vi "CANFD_Simple_Demo.vi"() -> ()   [LabVIEW 2014]
uses:
  TSMaster_API/CAN_CANFD_Function/Typedef/TLibCANFD.ctl
  <vilib>/Utility/miscctls.llb/LVPointTypeDef.ctl
  Utilities/Global/DLL_Path.vi
  Utilities/Typedef/Hardware_Subtype.ctl
  TSMaster_API/CAN_CANFD_Function/Typedef/TSCAN_CANFD_Configuration.ctl
  TSMaster_API/All_Control/Typedef/Hardware Type.ctl
panel:
  in  "DLL_Path":path=path "D:/Program Files (x86)/TOSUN/TSMaster/bin/TSMaster.dll"
  in  "Enable CH4":bool
  in  "Enable CH3":bool
  in  "Enable CH2":bool
  in  "Enable CH1":bool=TRUE
  out "Connect":bool
  in  "tab control":enum32{"CANFD1", "CANFD2", "CANFD3", "CANFD4"}(tab)
  in  "CH1  FD Frame":u8(ring) items=["Ordinary CAN Data", "FD CAN Data"]
  in  "CH1 Display Message Type":u16(ring)=1 items=["Only read received messages", "Receive&Send messages"]
  in  "CH1 Terminator":u16(ring)=1 items=["Disable", "Enable"]
  in  "CH1 Physical Channel":i32(ring) items=["CHN1", "CHN2", "CHN3", "CHN4", "CHN5", "CHN6", "CHN7", "CHN8", "CHN9", "CHN10", "CHN11", "CHN12", "CHN13", "CHN14", "CHN15", "CHN16", "CHN17", "CHN18", "CHN19", "CHN20", "CHN21", "CHN22", "CHN23", "CHN24", "CHN25", "CHN26", "CHN27", "CHN28", "CHN29", "CHN30", "CHN31", "CHN32"]
  in  "CH1 Application Logic Channel":i32(ring) items=["CHN1", "CHN2", "CHN3", "CHN4", "CHN5", "CHN6", "CHN7", "CHN8", "CHN9", "CHN10", "CHN11", "CHN12", "CHN13", "CHN14", "CHN15", "CHN16", "CHN17", "CHN18", "CHN19", "CHN20", "CHN21", "CHN22", "CHN23", "CHN24", "CHN25", "CHN26", "CHN27", "CHN28", "CHN29", "CHN30", "CHN31", "CHN32"]
  in  "CH1 Arbitration Field Baud Rate":sgl=500.0 format="%#_g k"
  in  "CH1 Data Field Baud Rate":sgl=2000.0 format="%#_g k"
  in  "CH1 Controller Type":i32(ring)=1 items=["lfdtCAN", "lfdtISOFDCAN", "lfdtNonISOFDFDCAN"]
  in  "CH1 Controller Working Mode":i32(ring) items=["lfdmNormal", "lfdmACKOff", "lfdmRestricted"]
  in  "CH1 Sending":bool
  in  "CH1ID":i32 format="%x"
  in  "CH1 Frame Format":u8(ring) items=["Standard Frame", "Extended Frame"]
  in  "CH1 Frame Type":u8(ring) items=["Data Frame", "Remote Frame", ""]
  in  "CH1SendData":u8[](array[numeric])=[0, 0, 0, 0, 0, 0, 0, 0, 0, 0, 0, 0, 0, 0, 0, 0, 0, 0, 0, 0, 0, 0, 0, 0, 0, 0, 0, 0, 0, 0, 0, 0, 0, 0, 0, 0, 0, 0, 0, 0, 0, 0, 0, 0, 0, 0, 0, 0, 0, 0, 0, 0, 0, 0, 0, 0, 0, 0, 0, 0, 0, 0, 0, 0, 0, 0, 0, 0, 0, 0, 0, 0, 0, 0, 0] format="%x"
  in  "CH1Data":i32(listbox)=-1
  in  "BRS":enum16{"Close", "Open"}(ring)
  in  "CANFD DLC":i32(ring)=15 caption="Data Length" items=["0", "1", "2", "3", "4", "5", "6", "7", "8", "12", "16", "20", "24", "32", "48", "64"]
  in  "Hardware Subtype":T1=enum."TC1016"
  in  "BRS 2":enum16{"Close", "Open"}(ring)
  in  "Hardware Subtype 2":T1=enum."TC1016"
  in  "CANFD DLC 2":i32(ring)=15 caption="Data Length" items=["0", "1", "2", "3", "4", "5", "6", "7", "8", "12", "16", "20", "24", "32", "48", "64"]
  in  "CH2  FD Frame":u8(ring) items=["Ordinary CAN Data", "FD CAN Data"]
  in  "CH2 Display Message Type":u16(ring)=1 items=["Rx", "Rx&Tx"]
  in  "CH2 Terminator":u16(ring)=1 items=["Disable", "Enable"]
  in  "CH2 Physical Channel":i32(ring)=1 items=["CHN1", "CHN2", "CHN3", "CHN4", "CHN5", "CHN6", "CHN7", "CHN8", "CHN9", "CHN10", "CHN11", "CHN12", "CHN13", "CHN14", "CHN15", "CHN16", "CHN17", "CHN18", "CHN19", "CHN20", "CHN21", "CHN22", "CHN23", "CHN24", "CHN25", "CHN26", "CHN27", "CHN28", "CHN29", "CHN30", "CHN31", "CHN32"]
  in  "CH2 Application Logic Channel":i32(ring)=1 items=["CHN1", "CHN2", "CHN3", "CHN4", "CHN5", "CHN6", "CHN7", "CHN8", "CHN9", "CHN10", "CHN11", "CHN12", "CHN13", "CHN14", "CHN15", "CHN16", "CHN17", "CHN18", "CHN19", "CHN20", "CHN21", "CHN22", "CHN23", "CHN24", "CHN25", "CHN26", "CHN27", "CHN28", "CHN29", "CHN30", "CHN31", "CHN32"]
  in  "CH2 Arbitration Field Baud Rate":sgl=500.0 format="%#_g k"
  in  "CH2 Data Field Baud Rate":sgl=2000.0 format="%#_g k"
  in  "CH2 Controller Type":i32(ring) items=["lfdtCAN", "lfdtISOFDCAN", "lfdtNonISOFDFDCAN"]
  in  "CH2 Controller Working Mode":i32(ring) items=["lfdmNormal", "lfdmACKOff", "lfdmRestricted"]
  in  "CH2 Sending":bool
  in  "CH2ID":i32 format="%x"
  in  "CH2 Frame Format":u8(ring) items=["Standard Frame", "Extended Frame"]
  in  "CH2 Frame Type":u8(ring) items=["Data Frame", "Remote Frame"]
  in  "CH2SendData":u8[](array[numeric])=[0, 0, 0, 0, 0, 0, 0, 0, 0, 0, 0, 0, 0, 0, 0, 0, 0, 0, 0, 0, 0, 0, 0, 0, 0, 0, 0, 0, 0, 0, 0, 0, 0, 0, 0, 0, 0, 0, 0, 0, 0, 0, 0, 0, 0, 0, 0, 0, 0, 0, 0, 0, 0, 0, 0, 0, 0, 0, 0, 0, 0, 0, 0, 0, 0, 0, 0, 0, 0, 0, 0, 0, 0, 0, 0, 0] format="%x"
  in  "CH2Data":i32(listbox)=-1
  in  "BRS 3":enum16{"Close", "Open"}(ring)
  in  "Hardware Subtype 3":T1=enum."TC1016"
  in  "CANFD DLC 3":i32(ring)=15 caption="Data Length" items=["0", "1", "2", "3", "4", "5", "6", "7", "8", "12", "16", "20", "24", "32", "48", "64"]
  in  "CH3 FD Frame":u8(ring) items=["Ordinary CAN Data", "FD CAN Data"]
  in  "CH3 Display Message Type":u16(ring)=1 items=["Rx", "Rx&Tx"]
  in  "CH Terminator":u16(ring)=1 items=["Disable", "Enable"]
  in  "CH3 Physical Channel":i32(ring)=2 items=["CHN1", "CHN2", "CHN3", "CHN4", "CHN5", "CHN6", "CHN7", "CHN8", "CHN9", "CHN10", "CHN11", "CHN12", "CHN13", "CHN14", "CHN15", "CHN16", "CHN17", "CHN18", "CHN19", "CHN20", "CHN21", "CHN22", "CHN23", "CHN24", "CHN25", "CHN26", "CHN27", "CHN28", "CHN29", "CHN30", "CHN31", "CHN32"]
  in  "CH3 Application Logic Channel":i32(ring)=2 items=["CHN1", "CHN2", "CHN3", "CHN4", "CHN5", "CHN6", "CHN7", "CHN8", "CHN9", "CHN10", "CHN11", "CHN12", "CHN13", "CHN14", "CHN15", "CHN16", "CHN17", "CHN18", "CHN19", "CHN20", "CHN21", "CHN22", "CHN23", "CHN24", "CHN25", "CHN26", "CHN27", "CHN28", "CHN29", "CHN30", "CHN31", "CHN32"]
  in  "CH3 Arbitration Field Baud Rate":sgl=500.0 format="%#_g k"
  in  "CH3 Data Field Baud Rate":sgl=2000.0 format="%#_g k"
  in  "CH3 Controller Type":i32(ring)=1 items=["lfdtCAN", "lfdtISOFDCAN", "lfdtNonISOFDFDCAN"]
  in  "CH3 Controller Working Mode":i32(ring) items=["lfdmNormal", "lfdmACKOff", "lfdmRestricted"]
  in  "CH3 Sending":bool
  in  "CH3ID":i32 format="%x"
  in  "CH3 Frame Format":u8(ring) items=["Standard Frame", "Extended Frame"]
  in  "CH3 Frame Type":u8(ring) items=["Data Frame", "Remote Frame"]
  in  "CH3SendData":u8[](array[numeric])=[0, 0, 0, 0, 0, 0, 0, 0, 0, 0, 0, 0, 0, 0, 0, 0, 0, 0, 0, 0, 0, 0, 0, 0, 0, 0, 0, 0, 0, 0, 0, 0, 0, 0, 0, 0, 0, 0, 0, 0, 0, 0, 0, 0, 0, 0, 0, 0, 0, 0, 0, 0, 0, 0, 0, 0, 0, 0, 0, 0, 0, 0, 0, 0, 0, 0, 0, 0, 0, 0, 0, 0, 0, 0, 0, 0] format="%x"
  in  "CH3Data":i32(listbox)=-1
  in  "BRS 4":enum16{"Close", "Open"}(ring)
  in  "Hardware Subtype 4":T1=enum."TC1016"
  in  "CANFD DLC 4":i32(ring)=15 caption="Data Length" items=["0", "1", "2", "3", "4", "5", "6", "7", "8", "12", "16", "20", "24", "32", "48", "64"]
  in  "CH4  FD Frame":u8(ring) items=["Ordinary CAN Data", "FD CAN Data"]
  in  "CH4 Display Message Type":u16(ring)=1 items=["Rx", "Rx&Tx"]
  in  "CH4 Terminator":u16(ring)=1 items=["Disable", "Enable"]
  in  "CH4 Physical Channel":i32(ring)=3 items=["CHN1", "CHN2", "CHN3", "CHN4", "CHN5", "CHN6", "CHN7", "CHN8", "CHN9", "CHN10", "CHN11", "CHN12", "CHN13", "CHN14", "CHN15", "CHN16", "CHN17", "CHN18", "CHN19", "CHN20", "CHN21", "CHN22", "CHN23", "CHN24", "CHN25", "CHN26", "CHN27", "CHN28", "CHN29", "CHN30", "CHN31", "CHN32"]
  in  "CH4 Application Logic Channel":i32(ring)=3 items=["CHN1", "CHN2", "CHN3", "CHN4", "CHN5", "CHN6", "CHN7", "CHN8", "CHN9", "CHN10", "CHN11", "CHN12", "CHN13", "CHN14", "CHN15", "CHN16", "CHN17", "CHN18", "CHN19", "CHN20", "CHN21", "CHN22", "CHN23", "CHN24", "CHN25", "CHN26", "CHN27", "CHN28", "CHN29", "CHN30", "CHN31", "CHN32"]
  in  "CH4 Arbitration Field Baud Rate":sgl=500.0 format="%#_g k"
  in  "CH4 Data Field Baud Rate":sgl=2000.0 format="%#_g k"
  in  "CH4 Controller Type":i32(ring)=1 items=["lfdtCAN", "lfdtISOFDCAN", "lfdtNonISOFDFDCAN"]
  in  "CH4 Controller Working Mode":i32(ring) items=["lfdmNormal", "lfdmACKOff", "lfdmRestricted"]
  in  "CH4 Sending":bool
  in  "CH4ID":i32 format="%x"
  in  "CH4 Frame Format":u8(ring) items=["Standard Frame", "Extended Frame"]
  in  "CH4 Frame Type":u8(ring) items=["Data Frame", "Remote Frame"]
  in  "CH4SendData":u8[](array[numeric])=[0, 0, 0, 0, 0, 0, 0, 0, 0, 0, 0, 0, 0, 0, 0, 0, 0, 0, 0, 0, 0, 0, 0, 0, 0, 0, 0, 0, 0, 0, 0, 0, 0, 0, 0, 0, 0, 0, 0, 0, 0, 0, 0, 0, 0, 0, 0, 0, 0, 0, 0, 0, 0, 0, 0, 0, 0, 0, 0, 0, 0, 0, 0, 0, 0, 0, 0, 0, 0, 0, 0, 0, 0, 0, 0, 0] format="%x"
  in  "CH4Data":i32(listbox)=-1
  in  "Number of channels used":u16(ring)=1 items=["1 Channel"=1, "2 Channels"=2, "3 Channels"=3, "4 Channels"=4, "5 Channels"=5]
  in  "Hardware on/off":bool
  in  "Exit":bool
  # "Standard Frame\nExtended Frame\nData Frame\nRemote Frame\nOrdinary CAN Data\nFD CAN Data"
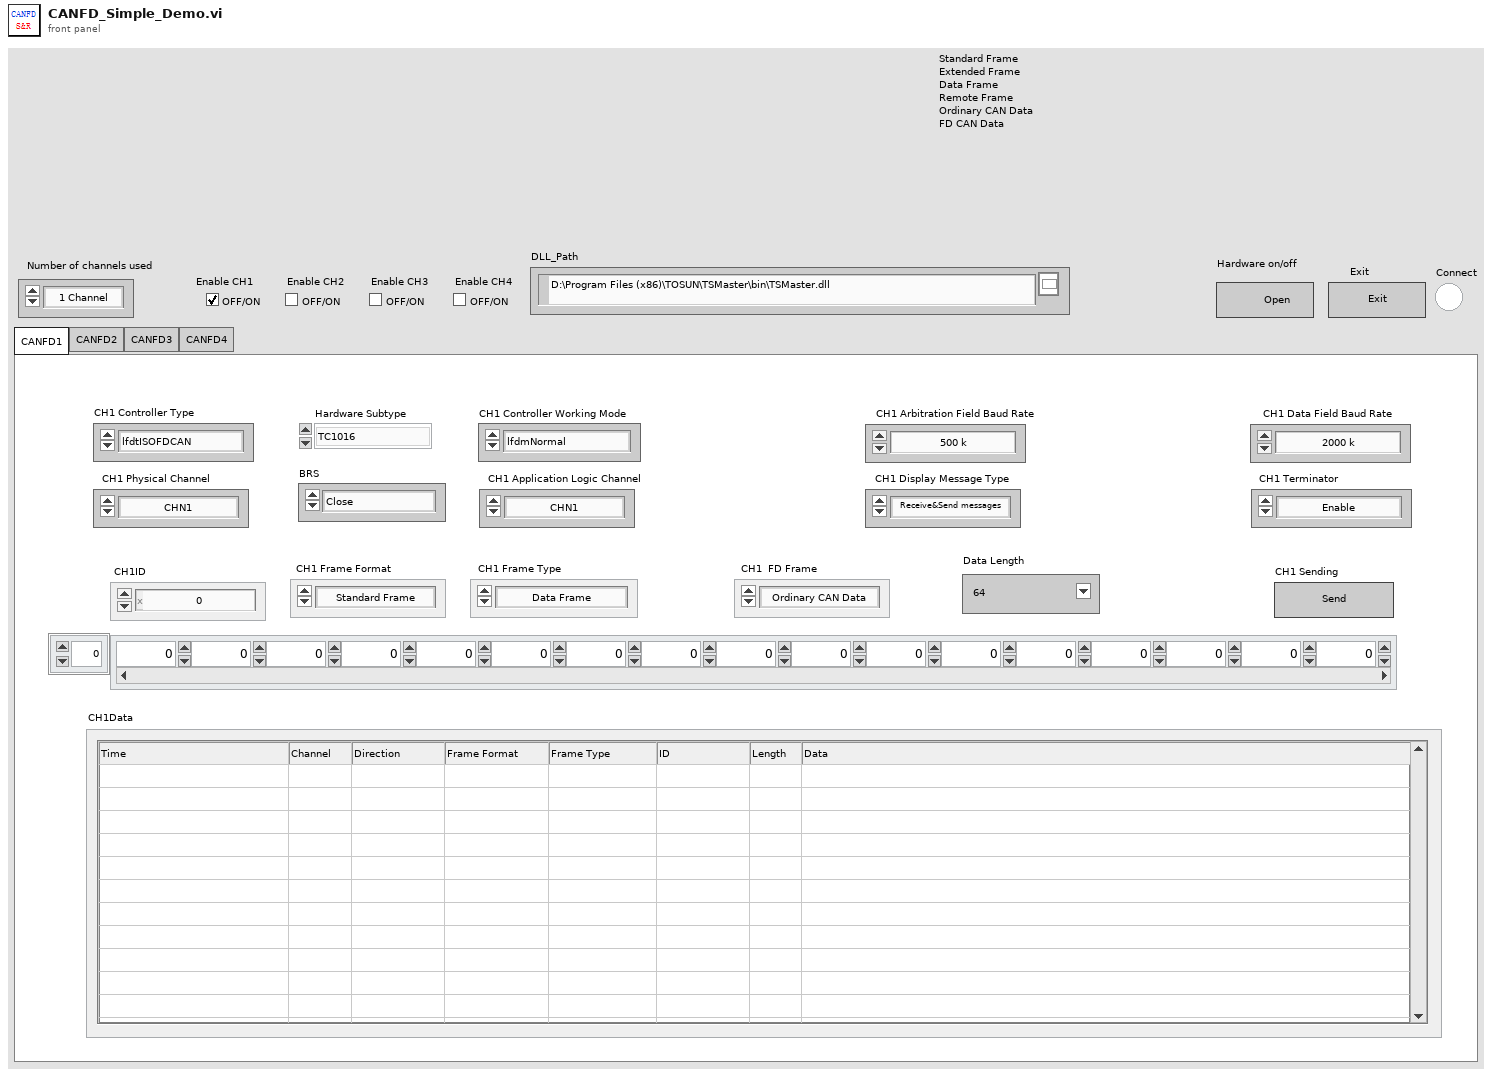
[diagram p1: front panel]
types:
  T1 = typedef "Hardware_Subtype.ctl" = enum16{"TS_UNKNOWN_DEVICE", "TSCAN_PRO", "TSCAN_Lite1", "TC1001", "TL1001", "TC1011", "TM5011", "TC1002", "TC1014", "TSCANFD2517", "TC1026", "TC1016", "TC1012", "TC1013", "TLog1002", "TC1034", "TC1018", "GW2116", "TC2115", "MP1013", "TC1113", "TC1114", "TP1013", "TC1017", "TP1018", "TF10XX", "TL1004_FD_4_LIN_2", "TE1051", "TP1051", "TP1034", "TTS9015", "TP1026", "TTS1026", "TTS1034", "TTS1018", "TL1011", "TTS1015_LiAuto", "TTS1013_LiAuto", "TTS1016Pro", "TC1054Pro", "TC1054", "TLog1038", "TO1013", "TC1034Pro", "TC1018Pro", "TC1038Pro", "TS_DEV_END"}
  T2 = typedef "LVPointTypeDef.ctl" = cluster{"Horizontal":i16, "Vertical":i16}
  T3 = cluster{"FIdxChn":u8, "FProperties":u8, "FDLC":u8, "FReserved":u8, "FIdentifier":i32, "FTimeUS":u64, "簇":cluster{"初始化的数组[0]":u8, "初始化的数组[1]":u8, "初始化的数组[2]":u8, "初始化的数组[3]":u8, "初始化的数组[4]":u8, "初始化的数组[5]":u8, "初始化的数组[6]":u8, "初始化的数组[7]":u8, "初始化的数组[8]":u8, "初始化的数组[9]":u8, "初始化的数组[10]":u8, "初始化的数组[11]":u8, "初始化的数组[12]":u8, "初始化的数组[13]":u8, "初始化的数组[14]":u8, "初始化的数组[15]":u8, "初始化的数组[16]":u8, "初始化的数组[17]":u8, "初始化的数组[18]":u8, "初始化的数组[19]":u8, "初始化的数组[20]":u8, "初始化的数组[21]":u8, "初始化的数组[22]":u8, "初始化的数组[23]":u8, "初始化的数组[24]":u8, "初始化的数组[25]":u8, "初始化的数组[26]":u8, "初始化的数组[27]":u8, "初始化的数组[28]":u8, "初始化的数组[29]":u8, "初始化的数组[30]":u8, "初始化的数组[31]":u8, "初始化的数组[32]":u8, "初始化的数组[33]":u8, "初始化的数组[34]":u8, "初始化的数组[35]":u8, "初始化的数组[36]":u8, "初始化的数组[37]":u8, "初始化的数组[38]":u8, "初始化的数组[39]":u8, "初始化的数组[40]":u8, "初始化的数组[41]":u8, "初始化的数组[42]":u8, "初始化的数组[43]":u8, "初始化的数组[44]":u8, "初始化的数组[45]":u8, "初始化的数组[46]":u8, "初始化的数组[47]":u8, "初始化的数组[48]":u8, "初始化的数组[49]":u8, "初始化的数组[50]":u8, "初始化的数组[51]":u8, "初始化的数组[52]":u8, "初始化的数组[53]":u8, "初始化的数组[54]":u8, "初始化的数组[55]":u8, "初始化的数组[56]":u8, "初始化的数组[57]":u8, "初始化的数组[58]":u8, "初始化的数组[59]":u8, "初始化的数组[60]":u8, "初始化的数组[61]":u8, "初始化的数组[62]":u8, "初始化的数组[63]":u8}}[]
  T4 = typedef "TLibCANFD.ctl" = cluster{"AIdxchn":u8, "AId":i32, "AIsStd":u8, "BRS":enum16{"Close", "Open"}, "AIsData":u8, "ADLC":i32, "AIsFD":enum16{"Classic CAN Message", "FD CAN Message"}, "FDatas":cluster{"Initialize array[0]":u8, "Initialize array[1]":u8, "Initialize array[2]":u8, "Initialize array[3]":u8, "Initialize array[4]":u8, "Initialize array[5]":u8, "Initialize array[6]":u8, "Initialize array[7]":u8, "Initialize array[8]":u8, "Initialize array[9]":u8, "Initialize array[10]":u8, "Initialize array[11]":u8, "Initialize array[12]":u8, "Initialize array[13]":u8, "Initialize array[14]":u8, "Initialize array[15]":u8, "Initialize array[16]":u8, "Initialize array[17]":u8, "Initialize array[18]":u8, "Initialize array[19]":u8, "Initialize array[20]":u8, "Initialize array[21]":u8, "Initialize array[22]":u8, "Initialize array[23]":u8, "Initialize array[24]":u8, "Initialize array[25]":u8, "Initialize array[26]":u8, "Initialize array[27]":u8, "Initialize array[28]":u8, "Initialize array[29]":u8, "Initialize array[30]":u8, "Initialize array[31]":u8, "Initialize array[32]":u8, "Initialize array[33]":u8, "Initialize array[34]":u8, "Initialize array[35]":u8, "Initialize array[36]":u8, "Initialize array[37]":u8, "Initialize array[38]":u8, "Initialize array[39]":u8, "Initialize array[40]":u8, "Initialize array[41]":u8, "Initialize array[42]":u8, "Initialize array[43]":u8, "Initialize array[44]":u8, "Initialize array[45]":u8, "Initialize array[46]":u8, "Initialize array[47]":u8, "Initialize array[48]":u8, "Initialize array[49]":u8, "Initialize array[50]":u8, "Initialize array[51]":u8, "Initialize array[52]":u8, "Initialize array[53]":u8, "Initialize array[54]":u8, "Initialize array[55]":u8, "Initialize array[56]":u8, "Initialize array[57]":u8, "Initialize array[58]":u8, "Initialize array[59]":u8, "Initialize array[60]":u8, "Initialize array[61]":u8, "Initialize array[62]":u8, "Initialize array[63]":u8}}
  T5 = cluster{"AIdxchn":u8, "AId":i32, "AIsStd":u8, "AIsData":u8, "ADLC":u8, "簇":cluster{"初始化的数组[0]":u8, "初始化的数组[1]":u8, "初始化的数组[2]":u8, "初始化的数组[3]":u8, "初始化的数组[4]":u8, "初始化的数组[5]":u8, "初始化的数组[6]":u8, "初始化的数组[7]":u8, "初始化的数组[8]":u8, "初始化的数组[9]":u8, "初始化的数组[10]":u8, "初始化的数组[11]":u8, "初始化的数组[12]":u8, "初始化的数组[13]":u8, "初始化的数组[14]":u8, "初始化的数组[15]":u8, "初始化的数组[16]":u8, "初始化的数组[17]":u8, "初始化的数组[18]":u8, "初始化的数组[19]":u8, "初始化的数组[20]":u8, "初始化的数组[21]":u8, "初始化的数组[22]":u8, "初始化的数组[23]":u8, "初始化的数组[24]":u8, "初始化的数组[25]":u8, "初始化的数组[26]":u8, "初始化的数组[27]":u8, "初始化的数组[28]":u8, "初始化的数组[29]":u8, "初始化的数组[30]":u8, "初始化的数组[31]":u8, "初始化的数组[32]":u8, "初始化的数组[33]":u8, "初始化的数组[34]":u8, "初始化的数组[35]":u8, "初始化的数组[36]":u8, "初始化的数组[37]":u8, "初始化的数组[38]":u8, "初始化的数组[39]":u8, "初始化的数组[40]":u8, "初始化的数组[41]":u8, "初始化的数组[42]":u8, "初始化的数组[43]":u8, "初始化的数组[44]":u8, "初始化的数组[45]":u8, "初始化的数组[46]":u8, "初始化的数组[47]":u8, "初始化的数组[48]":u8, "初始化的数组[49]":u8, "初始化的数组[50]":u8, "初始化的数组[51]":u8, "初始化的数组[52]":u8, "初始化的数组[53]":u8, "初始化的数组[54]":u8, "初始化的数组[55]":u8, "初始化的数组[56]":u8, "初始化的数组[57]":u8, "初始化的数组[58]":u8, "初始化的数组[59]":u8, "初始化的数组[60]":u8, "初始化的数组[61]":u8, "初始化的数组[62]":u8, "初始化的数组[63]":u8, "初始化的数组[64] ":u8}}
  T6 = cluster{"FIdxChn":u8, "FProperties":u8, "FDLC":u8, "FReserved":u8, "FIdentifier":i32, "FTimeUS":u64, "FData":cluster{"Data0":u8, "Data1":u8, "Data2":u8, "Data3":u8, "Data4":u8, "Data5":u8, "Data6":u8, "Data7":u8}}[]
  T7 = cluster{"FIdxChn":u8, "FProperties":u8, "FDLC":u8, "FReserved":u8, "FIdentifier":i32, "FTimeUS":u64, "Fdata":cluster{"初始化的数组[0]":u8, "初始化的数组[1]":u8, "初始化的数组[2]":u8, "初始化的数组[3]":u8, "初始化的数组[4]":u8, "初始化的数组[5]":u8, "初始化的数组[6]":u8, "初始化的数组[7]":u8, "初始化的数组[8]":u8, "初始化的数组[9]":u8, "初始化的数组[10]":u8, "初始化的数组[11]":u8, "初始化的数组[12]":u8, "初始化的数组[13]":u8, "初始化的数组[14]":u8, "初始化的数组[15]":u8, "初始化的数组[16]":u8, "初始化的数组[17]":u8, "初始化的数组[18]":u8, "初始化的数组[19]":u8, "初始化的数组[20]":u8, "初始化的数组[21]":u8, "初始化的数组[22]":u8, "初始化的数组[23]":u8, "初始化的数组[24]":u8, "初始化的数组[25]":u8, "初始化的数组[26]":u8, "初始化的数组[27]":u8, "初始化的数组[28]":u8, "初始化的数组[29]":u8, "初始化的数组[30]":u8, "初始化的数组[31]":u8, "初始化的数组[32]":u8, "初始化的数组[33]":u8, "初始化的数组[34]":u8, "初始化的数组[35]":u8, "初始化的数组[36]":u8, "初始化的数组[37]":u8, "初始化的数组[38]":u8, "初始化的数组[39]":u8, "初始化的数组[40]":u8, "初始化的数组[41]":u8, "初始化的数组[42]":u8, "初始化的数组[43]":u8, "初始化的数组[44]":u8, "初始化的数组[45]":u8, "初始化的数组[46]":u8, "初始化的数组[47]":u8, "初始化的数组[48]":u8, "初始化的数组[49]":u8, "初始化的数组[50]":u8, "初始化的数组[51]":u8, "初始化的数组[52]":u8, "初始化的数组[53]":u8, "初始化的数组[54]":u8, "初始化的数组[55]":u8, "初始化的数组[56]":u8, "初始化的数组[57]":u8, "初始化的数组[58]":u8, "初始化的数组[59]":u8, "初始化的数组[60]":u8, "初始化的数组[61]":u8, "初始化的数组[62]":u8, "初始化的数组[63]":u8}}[]
  T8 = typedef "TSCAN_CANFD_Configuration.ctl" = cluster{"Hardware Type":T9, "Hardware Subtype":T1, "AArbRateKbps":sgl, "AListenOnly":enum16{"Normal", "ListenOnly"}, "Int120Ohm":enum16{"Disable", "Enable"}, "EnableChannel":enum16{"Disable", "Enable"}, "AHwChannel":i32, "AAppChannel":i32, "ADataRateKbps":sgl, "AControllerType":i32, "AControllerMode":i32, "AldHW":i32}
  T9 = typedef "Hardware Type.ctl" = i32
  T10 = cluster{"CH1SendData[0]":u8, "CH1SendData[1]":u8, "CH1SendData[2]":u8, "CH1SendData[3]":u8, "CH1SendData[4]":u8, "CH1SendData[5]":u8, "CH1SendData[6]":u8, "CH1SendData[7]":u8, "CH1SendData[8]":u8, "CH1SendData[9]":u8, "CH1SendData[10]":u8, "CH1SendData[11]":u8, "CH1SendData[12]":u8, "CH1SendData[13]":u8, "CH1SendData[14]":u8, "CH1SendData[15]":u8, "CH1SendData[16]":u8, "CH1SendData[17]":u8, "CH1SendData[18]":u8, "CH1SendData[19]":u8, "CH1SendData[20]":u8, "CH1SendData[21]":u8, "CH1SendData[22]":u8, "CH1SendData[23]":u8, "CH1SendData[24]":u8, "CH1SendData[25]":u8, "CH1SendData[26]":u8, "CH1SendData[27]":u8, "CH1SendData[28]":u8, "CH1SendData[29]":u8, "CH1SendData[30]":u8, "CH1SendData[31]":u8, "CH1SendData[32]":u8, "CH1SendData[33]":u8, "CH1SendData[34]":u8, "CH1SendData[35]":u8, "CH1SendData[36]":u8, "CH1SendData[37]":u8, "CH1SendData[38]":u8, "CH1SendData[39]":u8, "CH1SendData[40]":u8, "CH1SendData[41]":u8, "CH1SendData[42]":u8, "CH1SendData[43]":u8, "CH1SendData[44]":u8, "CH1SendData[45]":u8, "CH1SendData[46]":u8, "CH1SendData[47]":u8, "CH1SendData[48]":u8, "CH1SendData[49]":u8, "CH1SendData[50]":u8, "CH1SendData[51]":u8, "CH1SendData[52]":u8, "CH1SendData[53]":u8, "CH1SendData[54]":u8, "CH1SendData[55]":u8, "CH1SendData[56]":u8, "CH1SendData[57]":u8, "CH1SendData[58]":u8, "CH1SendData[59]":u8, "CH1SendData[60]":u8, "CH1SendData[61]":u8, "CH1SendData[62]":u8, "CH1SendData[63]":u8}
  T11 = cluster{"CH2SendData[0]":u8, "CH2SendData[1]":u8, "CH2SendData[2]":u8, "CH2SendData[3]":u8, "CH2SendData[4]":u8, "CH2SendData[5]":u8, "CH2SendData[6]":u8, "CH2SendData[7]":u8, "CH2SendData[8]":u8, "CH2SendData[9]":u8, "CH2SendData[10]":u8, "CH2SendData[11]":u8, "CH2SendData[12]":u8, "CH2SendData[13]":u8, "CH2SendData[14]":u8, "CH2SendData[15]":u8, "CH2SendData[16]":u8, "CH2SendData[17]":u8, "CH2SendData[18]":u8, "CH2SendData[19]":u8, "CH2SendData[20]":u8, "CH2SendData[21]":u8, "CH2SendData[22]":u8, "CH2SendData[23]":u8, "CH2SendData[24]":u8, "CH2SendData[25]":u8, "CH2SendData[26]":u8, "CH2SendData[27]":u8, "CH2SendData[28]":u8, "CH2SendData[29]":u8, "CH2SendData[30]":u8, "CH2SendData[31]":u8, "CH2SendData[32]":u8, "CH2SendData[33]":u8, "CH2SendData[34]":u8, "CH2SendData[35]":u8, "CH2SendData[36]":u8, "CH2SendData[37]":u8, "CH2SendData[38]":u8, "CH2SendData[39]":u8, "CH2SendData[40]":u8, "CH2SendData[41]":u8, "CH2SendData[42]":u8, "CH2SendData[43]":u8, "CH2SendData[44]":u8, "CH2SendData[45]":u8, "CH2SendData[46]":u8, "CH2SendData[47]":u8, "CH2SendData[48]":u8, "CH2SendData[49]":u8, "CH2SendData[50]":u8, "CH2SendData[51]":u8, "CH2SendData[52]":u8, "CH2SendData[53]":u8, "CH2SendData[54]":u8, "CH2SendData[55]":u8, "CH2SendData[56]":u8, "CH2SendData[57]":u8, "CH2SendData[58]":u8, "CH2SendData[59]":u8, "CH2SendData[60]":u8, "CH2SendData[61]":u8, "CH2SendData[62]":u8, "CH2SendData[63]":u8}
  T12 = cluster{"CH3SendData[0]":u8, "CH3SendData[1]":u8, "CH3SendData[2]":u8, "CH3SendData[3]":u8, "CH3SendData[4]":u8, "CH3SendData[5]":u8, "CH3SendData[6]":u8, "CH3SendData[7]":u8, "CH3SendData[8]":u8, "CH3SendData[9]":u8, "CH3SendData[10]":u8, "CH3SendData[11]":u8, "CH3SendData[12]":u8, "CH3SendData[13]":u8, "CH3SendData[14]":u8, "CH3SendData[15]":u8, "CH3SendData[16]":u8, "CH3SendData[17]":u8, "CH3SendData[18]":u8, "CH3SendData[19]":u8, "CH3SendData[20]":u8, "CH3SendData[21]":u8, "CH3SendData[22]":u8, "CH3SendData[23]":u8, "CH3SendData[24]":u8, "CH3SendData[25]":u8, "CH3SendData[26]":u8, "CH3SendData[27]":u8, "CH3SendData[28]":u8, "CH3SendData[29]":u8, "CH3SendData[30]":u8, "CH3SendData[31]":u8, "CH3SendData[32]":u8, "CH3SendData[33]":u8, "CH3SendData[34]":u8, "CH3SendData[35]":u8, "CH3SendData[36]":u8, "CH3SendData[37]":u8, "CH3SendData[38]":u8, "CH3SendData[39]":u8, "CH3SendData[40]":u8, "CH3SendData[41]":u8, "CH3SendData[42]":u8, "CH3SendData[43]":u8, "CH3SendData[44]":u8, "CH3SendData[45]":u8, "CH3SendData[46]":u8, "CH3SendData[47]":u8, "CH3SendData[48]":u8, "CH3SendData[49]":u8, "CH3SendData[50]":u8, "CH3SendData[51]":u8, "CH3SendData[52]":u8, "CH3SendData[53]":u8, "CH3SendData[54]":u8, "CH3SendData[55]":u8, "CH3SendData[56]":u8, "CH3SendData[57]":u8, "CH3SendData[58]":u8, "CH3SendData[59]":u8, "CH3SendData[60]":u8, "CH3SendData[61]":u8, "CH3SendData[62]":u8, "CH3SendData[63]":u8}
  T13 = cluster{"CH4SendData[0]":u8, "CH4SendData[1]":u8, "CH4SendData[2]":u8, "CH4SendData[3]":u8, "CH4SendData[4]":u8, "CH4SendData[5]":u8, "CH4SendData[6]":u8, "CH4SendData[7]":u8, "CH4SendData[8]":u8, "CH4SendData[9]":u8, "CH4SendData[10]":u8, "CH4SendData[11]":u8, "CH4SendData[12]":u8, "CH4SendData[13]":u8, "CH4SendData[14]":u8, "CH4SendData[15]":u8, "CH4SendData[16]":u8, "CH4SendData[17]":u8, "CH4SendData[18]":u8, "CH4SendData[19]":u8, "CH4SendData[20]":u8, "CH4SendData[21]":u8, "CH4SendData[22]":u8, "CH4SendData[23]":u8, "CH4SendData[24]":u8, "CH4SendData[25]":u8, "CH4SendData[26]":u8, "CH4SendData[27]":u8, "CH4SendData[28]":u8, "CH4SendData[29]":u8, "CH4SendData[30]":u8, "CH4SendData[31]":u8, "CH4SendData[32]":u8, "CH4SendData[33]":u8, "CH4SendData[34]":u8, "CH4SendData[35]":u8, "CH4SendData[36]":u8, "CH4SendData[37]":u8, "CH4SendData[38]":u8, "CH4SendData[39]":u8, "CH4SendData[40]":u8, "CH4SendData[41]":u8, "CH4SendData[42]":u8, "CH4SendData[43]":u8, "CH4SendData[44]":u8, "CH4SendData[45]":u8, "CH4SendData[46]":u8, "CH4SendData[47]":u8, "CH4SendData[48]":u8, "CH4SendData[49]":u8, "CH4SendData[50]":u8, "CH4SendData[51]":u8, "CH4SendData[52]":u8, "CH4SendData[53]":u8, "CH4SendData[54]":u8, "CH4SendData[55]":u8, "CH4SendData[56]":u8, "CH4SendData[57]":u8, "CH4SendData[58]":u8, "CH4SendData[59]":u8, "CH4SendData[60]":u8, "CH4SendData[61]":u8, "CH4SendData[62]":u8, "CH4SendData[63]":u8}
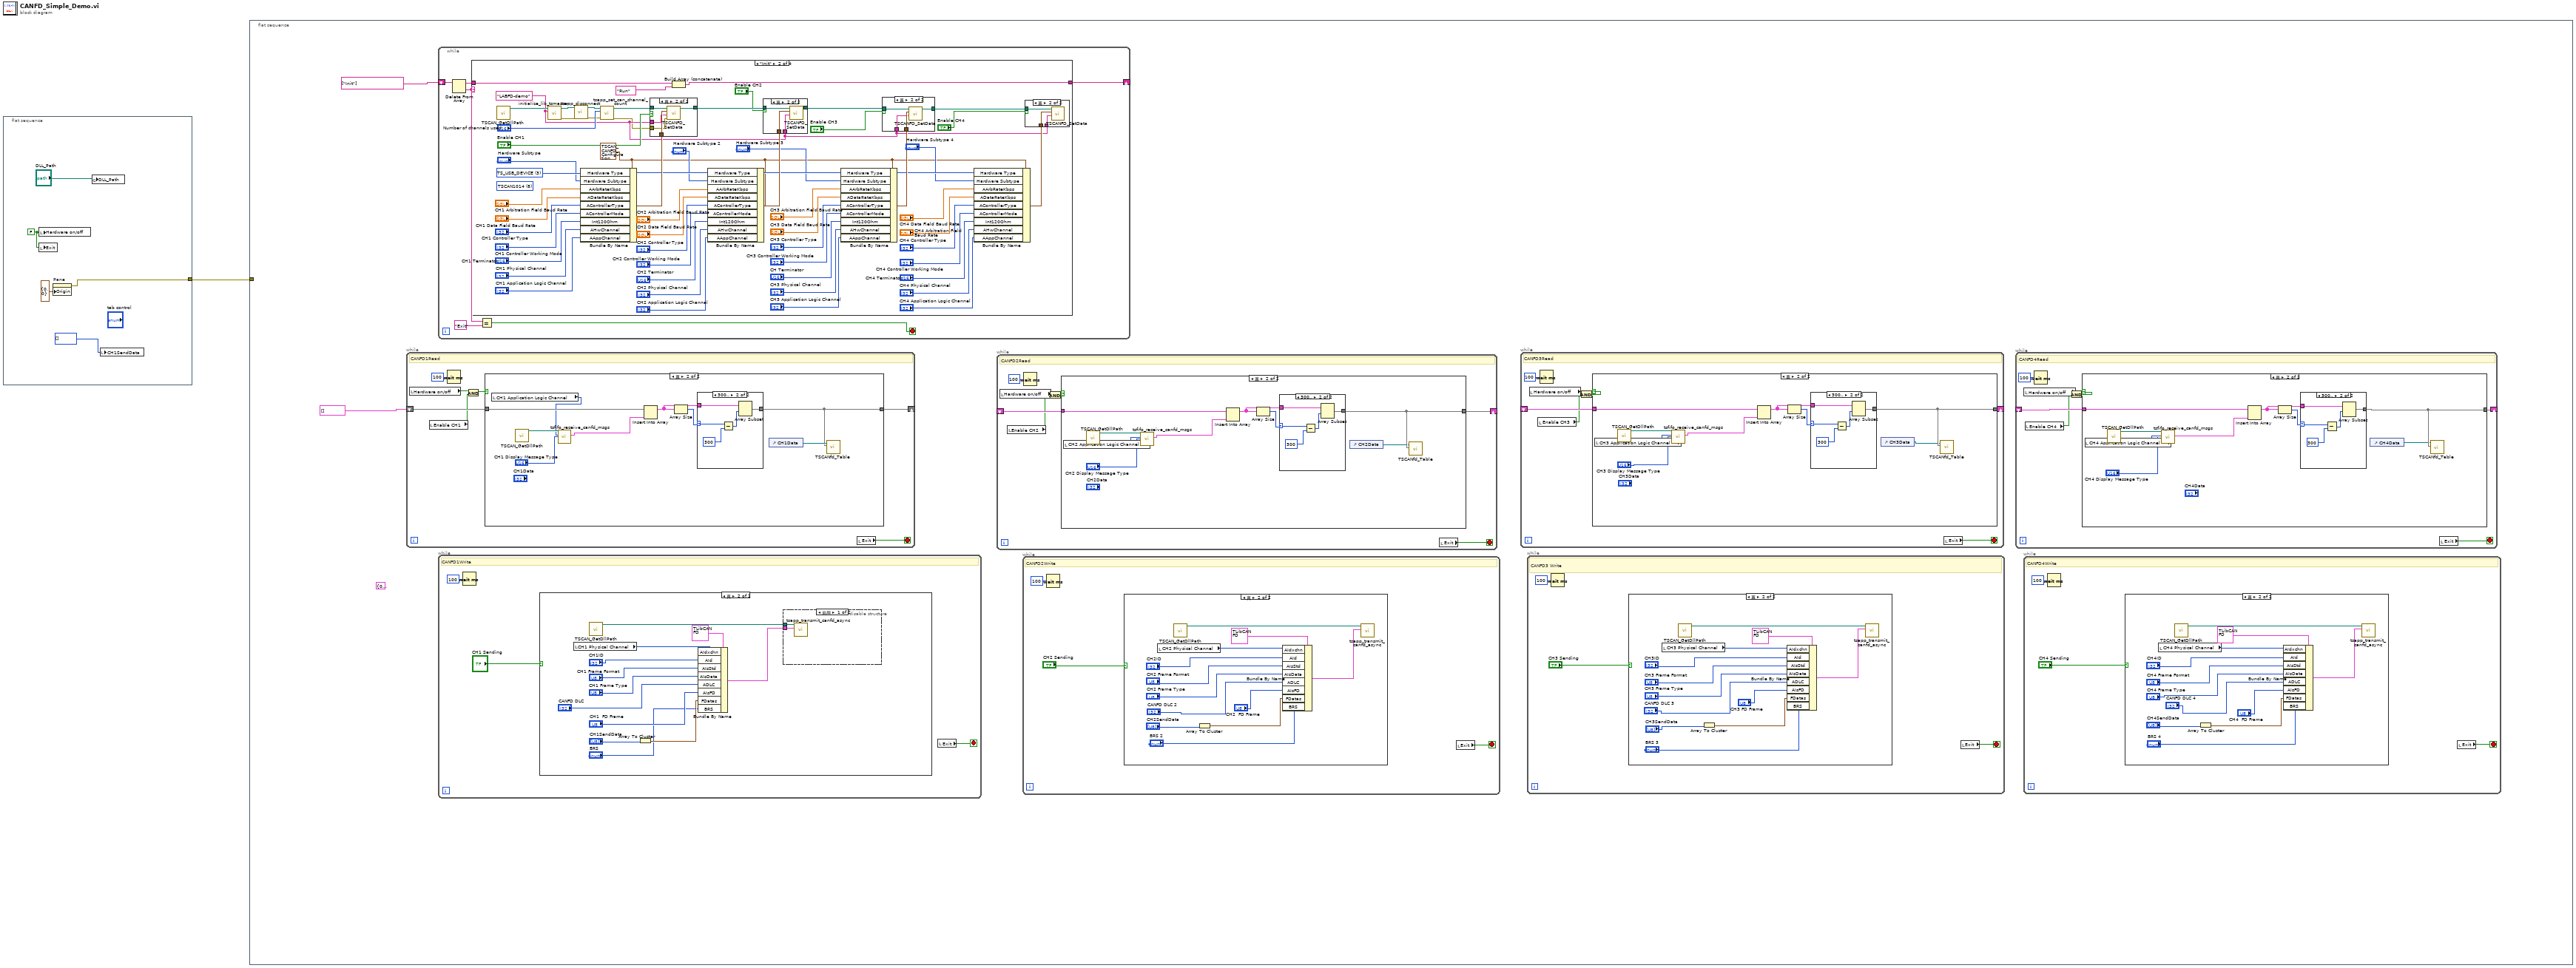
[diagram p0: block diagram]
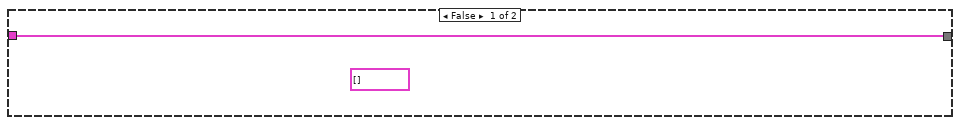
[diagram p3: hidden frame]
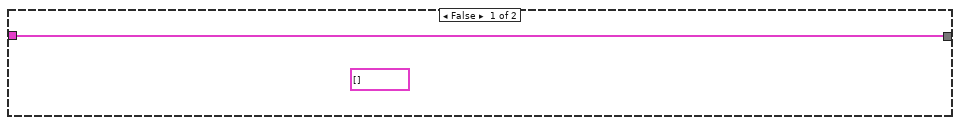
[diagram p6: hidden frame]
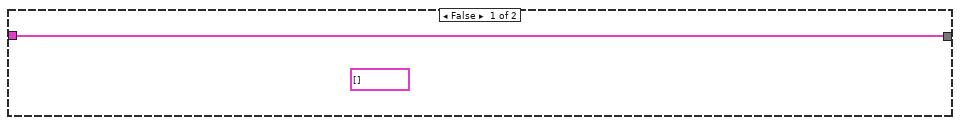
[diagram p9: hidden frame]
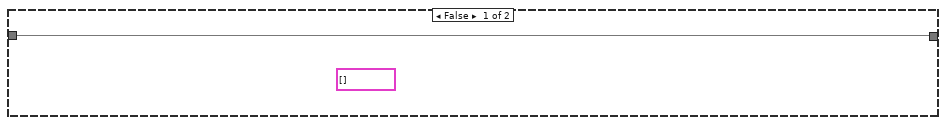
[diagram p13: hidden frame]
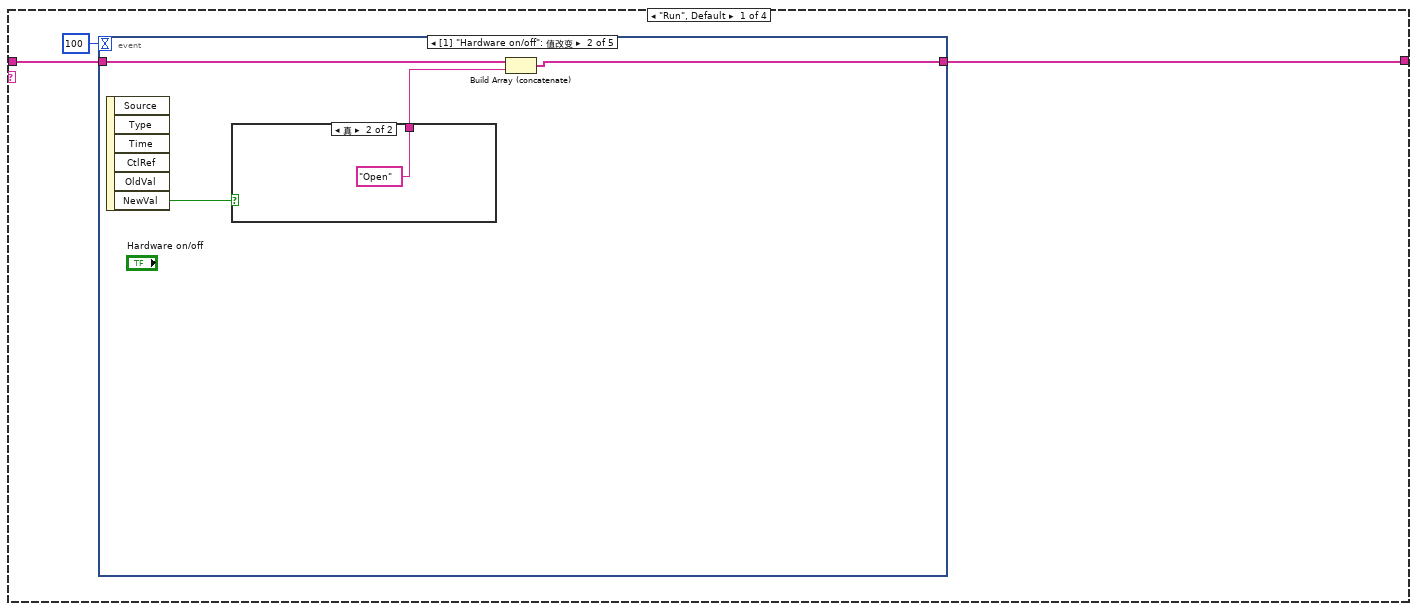
[diagram p15: hidden frame]
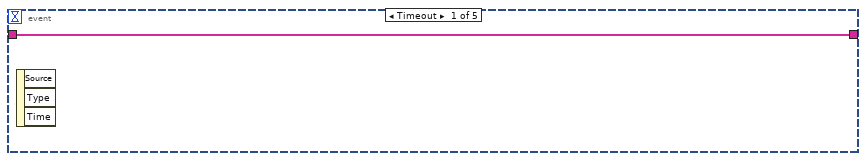
[diagram p16: hidden frame]
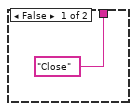
[diagram p17: hidden frame]
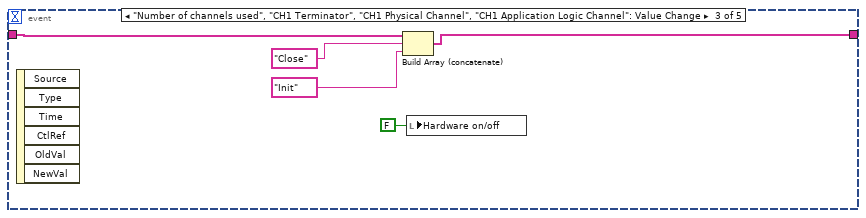
[diagram p18: hidden frame]
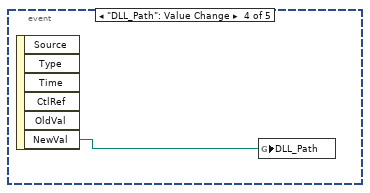
[diagram p19: hidden frame]
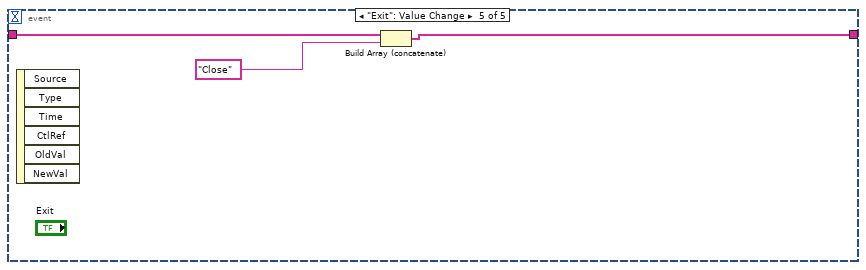
[diagram p20: hidden frame]
diagram:
  n1 = flat-sequence {
    tunnel: [w3] -> w1
    frame #0 {
      w6 = FALSE ("硬件启闭")
      n2 = local write "Hardware on/off"(w6) -> ()
      n3 = local write "Exit"(w6) -> ()
      n4 = property on="Pane" class="Pane"("Origin"=T2 {"Horizontal"=0, "Vertical"=0} ("原点")) -> (error out=w3:errorcluster)  [unwired: 2 in, 1 out]
      n5 = global write "DLL_Path.vi" "DLL_Path"("DLL_Path") -> ()
      n6 = local write "CH1SendData"(u8[] []) -> ()
    }
  }
  n7 = flat-sequence {
    tunnel: w1 -> [_]
    frame #0 {
      (unwired) T5 {"AIdxchn"=0, "AId"=0, "AIsStd"=0, "AIsData"=0, "ADLC"=0, "簇"={"初始化的数组[0]"=0, "初始化的数组[1]"=0, "初始化的数组[2]"=0, "初始化的数组[3]"=0, "初始化的数组[4]"=0, "初始化的数组[5]"=0, "初始化的数组[6]"=0, "初始化的数组[7]"=0, "初始化的数组[8]"=0, "初始化的数组[9]"=0, "初始化的数组[10]"=0, "初始化的数组[11]"=0, "初始化的数组[12]"=0, "初始化的数组[13]"=0, "初始化的数组[14]"=0, "初始化的数组[15]"=0, "初始化的数组[16]"=0, "初始化的数组[17]"=0, "初始化的数组[18]"=0, "初始化的数组[19]"=0, "初始化的数组[20]"=0, "初始化的数组[21]"=0, "初始化的数组[22]"=0, "初始化的数组[23]"=0, "初始化的数组[24]"=0, "初始化的数组[25]"=0, "初始化的数组[26]"=0, "初始化的数组[27]"=0, "初始化的数组[28]"=0, "初始化的数组[29]"=0, "初始化的数组[30]"=0, "初始化的数组[31]"=0, "初始化的数组[32]"=0, "初始化的数组[33]"=0, "初始化的数组[34]"=0, "初始化的数组[35]"=0, "初始化的数组[36]"=0, "初始化的数组[37]"=0, "初始化的数组[38]"=0, "初始化的数组[39]"=0, "初始化的数组[40]"=0, "初始化的数组[41]"=0, "初始化的数组[42]"=0, "初始化的数组[43]"=0, "初始化的数组[44]"=0, "初始化的数组[45]"=0, "初始化的数组[46]"=0, "初始化的数组[47]"=0, "初始化的数组[48]"=0, "初始化的数组[49]"=0, "初始化的数组[50]"=0, "初始化的数组[51]"=0, "初始化的数组[52]"=0, "初始化的数组[53]"=0, "初始化的数组[54]"=0, "初始化的数组[55]"=0, "初始化的数组[56]"=0, "初始化的数组[57]"=0, "初始化的数组[58]"=0, "初始化的数组[59]"=0, "初始化的数组[60]"=0, "初始化的数组[61]"=0, "初始化的数组[62]"=0, "初始化的数组[63]"=0, "初始化的数组[64] "=0}} ("TCAN 2")
      n8 = while {
        shift-right: [w143] -> _
        shift-left: T3 [] ("y") -> [w144]
        stop <- w146 stop-if-true
        # "CANFD1Read"
        n9 = local read "Hardware on/off"() -> (w142:bool)
        n10 = local read "Enable CH1"() -> (w141:bool)
        n11 = Wait (ms)(milliseconds to wait=u32 100 ("等待时间（毫秒）")) -> ()  [unwired: 1 out]
        n12 = And(x=w142, y=w141) -> (x .and. y?=w140:bool)
        n13 = case shown="真" w140 {
          tunnel: [w147 w149] -> w143
          tunnel: w144 -> [w147 w156]
          frame False {
            (unwired) T6 [] ("数组")
          }
          frame True {
            n14 = local read "CH1 Application Logic Channel"() -> (w152:i32)
            n15 = call "TSCAN_GetDllPath.vi"() -> ("DllPath"=w153:path)  [unwired: 11 in]
            n16 = call "tsfifo_receive_canfd_msgs.vi"("Display message type"="CH1 Display Message Type", "AAPPChannel"=w152, "Path"=w153) -> ("ACANMsgBuffer"=w148:T7)  [unwired: 4 in, 3 out]
            n17 = Insert Into Array(array=w156, new element=w148) -> (w154:T3)  [unwired: 1 in]
            n18 = Array Size(array=w154) -> (size(s)=w155:i32)
            n19 = case shown="300.." w155 {
              selector: w155 -> [_ w162]
              tunnel: [w157 w160] -> w149
              tunnel: w154 -> [w157 w158]
              frame 0, Default {
              }
              frame 300.. {
                n20 = Subtract(x=w162, y=300) -> (x-y=w159:i32)
                n21 = Array Subset(array=w158, index=w159) -> (w160:T3)  [unwired: 1 in]
              }
            }
            n22 = control-ref of="CH1Data"() -> (w150:refnum<vi>)
            n23 = call "TSCANfd_Table.vi"("Messages"=w149, "MCListbox reference handle"=w150) -> ()  [unwired: 10 in]
          }
        }
        n24 = local read "Exit"() -> (w146:bool)
      }
      n25 = while {
        shift-right: [w166] -> _
        shift-left: string[] ["Init"] -> [w168]
        stop <- w163 stop-if-true
        n26 = Delete From Array(array=w168) -> (deleted portion=w165:string, array with subset deleted=w167:string[])  [unwired: 2 in]
        n27 = case shown="\"Init\"" w165 {
          tunnel: w167 -> [w170 w239 w268 w274]
          tunnel: [w169 w238 w267 w275] -> w166
          frame "Run", Default {
            n28 = event shown="[1] \"Hardware on/off\": 值改变" {
              selector: _ -> [_ _ _ _ _]
              dyn-events: _ -> [_ _ _ _ _]
              timeout: 100 -> [_ _ _ _ _]
              tunnel: w170 -> [w172 w176 w183 _ w186]
              tunnel: [w172 w175 w181 _ w185] -> w169
              event Timeout {
                n29 = event-data() -> ()  [unwired: 1 in, 3 out]
              }
              event "Hardware on/off": Value Change {
                n30 = event-data() -> ("NewVal"=w174:bool)  [unwired: 1 in, 5 out]
                n31 = case shown="真" w174 {
                  tunnel: ["Close" "Open"] -> w173
                  frame False {
                  }
                  frame True {
                  }
                }
                n32 = Build Array (concatenate)(w176, w173) -> (w175:string[])
              }
              event "Number of channels used", "CH1 Terminator", "CH1 Physical Channel", "CH1 Application Logic Channel": Value Change {
                n33 = event-data() -> ()  [unwired: 1 in, 6 out]
                n34 = Build Array (concatenate)(w183, "Close", "Init") -> (w181:string[])
                n35 = local write "Hardware on/off"(FALSE ("硬件启闭")) -> ()
              }
              event "DLL_Path": Value Change {
                n36 = event-data() -> ("NewVal"=w184:path)  [unwired: 1 in, 5 out]
                n37 = global write "DLL_Path.vi" "DLL_Path"(w184) -> ()
              }
              event "Exit": Value Change {
                n38 = event-data() -> ()  [unwired: 1 in, 6 out]
                n39 = Build Array (concatenate)(w186, "Close") -> (w185:string[])
              }
            }
          }
          frame "Init" {
            w192 = T8 {"Hardware Type"=8, "Hardware Subtype"=enum."TC1016", "AArbRateKbps"=250.0, "AListenOnly"=enum."Normal", "Int120Ohm"=enum."Enable", "EnableChannel"=enum."Enable", "AHwChannel"=0, "AAppChannel"=0, "ADataRateKbps"=250.0, "AControllerType"=0, "AControllerMode"=0, "AldHW"=0} ("CANFD Configuration")
            w191 = "LABFD-demo" ("AppName")
            (unwired) 8 items=["BUS_UNKNOWN_TYPE", "TSCAN_PRO_4", "TSCAN_LITE_2", "TSCANMini", "TSLinMini", "TSCANFDmini", "TSCAN_LIN_IO_2", "TSCAN_LITE_2", "TSCAN1014", "TSCAN_FD_Mini_1"] ("硬件型号")
            w203 = 3 items=["BUS_UNKNOWN_TYPE", "TS_TCP_DEVICE", "XL_USB_DEVICE", "TS_USB_DEVICE", "PEAK_USB_DEVICE", "KVASER_USB_DEVICE", "ZLG_USB_DEVICE", "ICS_USB_DEVICE", "TS_TC1005_DEVICE"] ("硬件类型")
            n40 = call "TSCAN_GetDllPath.vi"() -> ("DllPath"=w242:path)  [unwired: 11 in]
            n41 = call "initialize_lib_tsmaster.vi"("AppName"=w191, "Path input"=w242) -> ("error output"=w190:errorcluster, "Path output"=w243:path)  [unwired: 8 in]
            n42 = call "tsapp_disconnect.vi"("error in (no error)"=w190, "Path"=w243) -> ("error output"=w189:errorcluster, "Path output"=w244:path)  [unwired: 7 in, 1 out]
            n43 = Bundle By Name(cluster=w192, "Hardware Type"=w203, "Hardware Subtype"="Hardware Subtype", "AArbRateKbps"="CH1 Arbitration Field Baud Rate", "ADataRateKbps"="CH1 Data Field Baud Rate", "AControllerType"="CH1 Controller Type", "AControllerMode"="CH1 Controller Working Mode", "Int120Ohm"="CH1 Terminator", "AHwChannel"="CH1 Physical Channel", "AAppChannel"="CH1 Application Logic Channel") -> (w229:T8)
            n44 = call "tsapp_set_can_channel_count.vi"("error in (no error)"=w189, "Aount"="Number of channels used", "Path"=w244) -> ("error out"=w188:errorcluster, "Path output"=w237:path)  [unwired: 6 in, 1 out]
            n45 = case shown="真" "Enable CH1" {
              tunnel: w237 -> [w258 w263]
              tunnel: w229 -> [_ w262]
              tunnel: [w258 w261] -> w228
              tunnel: w191 -> [_ w260]
              tunnel: w188 -> [_ w259]
              frame False {
              }
              frame True {
                n46 = call "TSCANFD_SetData.vi"("ERROR IN"=w259, "AppName"=w260, "CANFD Configuration"=w262, "PATH"=w263) -> ("PATH OUT"=w261:path)  [unwired: 4 in, 3 out]
              }
            }
            n47 = Build Array (concatenate)(w239, "Run") -> (w238:string[])
            n48 = Bundle By Name(cluster=w192, "Hardware Type"=w203, "Hardware Subtype"="Hardware Subtype 2", "AArbRateKbps"="CH2 Arbitration Field Baud Rate", "ADataRateKbps"="CH2 Data Field Baud Rate", "AControllerType"="CH2 Controller Type", "AControllerMode"="CH2 Controller Working Mode", "Int120Ohm"="CH2 Terminator", "AHwChannel"="CH2 Physical Channel", "AAppChannel"="CH2 Application Logic Channel") -> (w224:T8)
            n49 = case shown="真" "Enable CH2" {
              tunnel: w224 -> [_ w257]
              tunnel: w228 -> [w253 w256]
              tunnel: [w253 w255] -> w216
              tunnel: w191 -> [_ w254]
              frame False {
              }
              frame True {
                n50 = call "TSCANFD_SetData.vi"("AppName"=w254, "CANFD Configuration"=w257, "PATH"=w256) -> ("PATH OUT"=w255:path)  [unwired: 5 in, 3 out]
              }
            }
            n51 = Bundle By Name(cluster=w192, "Hardware Type"=w203, "Hardware Subtype"="Hardware Subtype 3", "AArbRateKbps"="CH3 Arbitration Field Baud Rate", "ADataRateKbps"="CH3 Data Field Baud Rate", "AControllerType"="CH3 Controller Type", "AControllerMode"="CH3 Controller Working Mode", "Int120Ohm"="CH Terminator", "AHwChannel"="CH3 Physical Channel", "AAppChannel"="CH3 Application Logic Channel") -> (w213:T8)
            n52 = case shown="真" "Enable CH3" {
              tunnel: w216 -> [w248 w252]
              tunnel: [w248 w251] -> w215
              tunnel: w213 -> [_ w250]
              tunnel: w191 -> [_ w249]
              frame False {
              }
              frame True {
                n53 = call "TSCANFD_SetData.vi"("AppName"=w249, "CANFD Configuration"=w250, "PATH"=w252) -> ("PATH OUT"=w251:path)  [unwired: 5 in, 3 out]
              }
            }
            n54 = Bundle By Name(cluster=w192, "Hardware Type"=w203, "Hardware Subtype"="Hardware Subtype 4", "AArbRateKbps"="CH4 Data Field Baud Rate", "ADataRateKbps"="CH4 Arbitration Field Baud Rate", "AControllerType"="CH4 Controller Type", "AControllerMode"="CH4 Controller Working Mode", "Int120Ohm"="CH4 Terminator", "AHwChannel"="CH4 Physical Channel", "AAppChannel"="CH4 Application Logic Channel") -> (w212:T8)
            n55 = case shown="真" "Enable CH4" {
              tunnel: w212 -> [_ w247]
              tunnel: w215 -> [_ w246]
              tunnel: w191 -> [_ w245]
              frame False {
              }
              frame True {
                n56 = call "TSCANFD_SetData.vi"("AppName"=w245, "CANFD Configuration"=w247, "PATH"=w246) -> ()  [unwired: 5 in, 4 out]
              }
            }
          }
          frame "Open" {
            n57 = call "TSCAN_GetDllPath.vi"() -> ("DllPath"=w264:path)  [unwired: 11 in]
            n58 = call "tsapp_connect.vi"("Path"=w264) -> ("retuen"=w266:i32, "Path output"=w270:path)  [unwired: 8 in, 1 out]
            n59 = Build Array (concatenate)(w268, "Run") -> (w267:string[])
            n60 = Equal To 0?(x=w266) -> (x = 0?=→"Connect":bool)
            n61 = call "tsfifo_enable_receive_fifo.vi"("Path"=w270) -> ()  [unwired: 9 in, 2 out]
          }
          frame "Close" {
            n62 = call "TSCAN_GetDllPath.vi"() -> ("DllPath"=w273:path)  [unwired: 11 in]
            n63 = local write "Connect"(FALSE ("通讯")) -> ()
            n64 = call "finalize_lib_tsmaster.vi"("Path"=w273) -> ("error out"=w272:errorcluster)  [unwired: 9 in, 1 out]
            n65 = local read "Exit"() -> (w276:bool)
            n66 = case shown="假" w276 {
              tunnel: [w277 w281] -> w275
              tunnel: w274 -> [w278 w280]
              tunnel: w272 -> [_ _]
              frame False {
                n67 = Build Array (concatenate)(w278, "Run") -> (w277:string[])
              }
              frame True {
                n68 = Build Array (concatenate)(w280, "Exit") -> (w281:string[])
              }
            }
          }
        }
        n69 = Equal?(x=w165, y="Exit") -> (x = y?=w163:bool)
      }
      n70 = while {
        stop <- w125 stop-if-true
        # "CANFD1Write"
        n71 = Wait (ms)(milliseconds to wait=u32 100 ("等待时间（毫秒）")) -> ()  [unwired: 1 out]
        n72 = case shown="真" "CH1 Sending" {
          frame False {
          }
          frame True {
            n73 = local read "CH1 Physical Channel"() -> (w127:i32)
            n74 = call "TSCAN_GetDllPath.vi"() -> ("DllPath"=w131:path)  [unwired: 11 in]
            n75 = Array To Cluster(array="CH1SendData") -> (cluster=w133:T10)
            n76 = Bundle By Name(cluster=T4 {"AIdxchn"=0, "AId"=0, "AIsStd"=0, "BRS"=enum."Close", "AIsData"=0, "ADLC"=0, "AIsFD"=enum."Classic CAN Message", "FDatas"={"Initialize array[0]"=0, "Initialize array[1]"=0, "Initialize array[2]"=0, "Initialize array[3]"=0, "Initialize array[4]"=0, "Initialize array[5]"=0, "Initialize array[6]"=0, "Initialize array[7]"=0, "Initialize array[8]"=0, "Initialize array[9]"=0, "Initialize array[10]"=0, "Initialize array[11]"=0, "Initialize array[12]"=0, "Initialize array[13]"=0, "Initialize array[14]"=0, "Initialize array[15]"=0, "Initialize array[16]"=0, "Initialize array[17]"=0, "Initialize array[18]"=0, "Initialize array[19]"=0, "Initialize array[20]"=0, "Initialize array[21]"=0, "Initialize array[22]"=0, "Initialize array[23]"=0, "Initialize array[24]"=0, "Initialize array[25]"=0, "Initialize array[26]"=0, "Initialize array[27]"=0, "Initialize array[28]"=0, "Initialize array[29]"=0, "Initialize array[30]"=0, "Initialize array[31]"=0, "Initialize array[32]"=0, "Initialize array[33]"=0, "Initialize array[34]"=0, "Initialize array[35]"=0, "Initialize array[36]"=0, "Initialize array[37]"=0, "Initialize array[38]"=0, "Initialize array[39]"=0, "Initialize array[40]"=0, "Initialize array[41]"=0, "Initialize array[42]"=0, "Initialize array[43]"=0, "Initialize array[44]"=0, "Initialize array[45]"=0, "Initialize array[46]"=0, "Initialize array[47]"=0, "Initialize array[48]"=0, "Initialize array[49]"=0, "Initialize array[50]"=0, "Initialize array[51]"=0, "Initialize array[52]"=0, "Initialize array[53]"=0, "Initialize array[54]"=0, "Initialize array[55]"=0, "Initialize array[56]"=0, "Initialize array[57]"=0, "Initialize array[58]"=0, "Initialize array[59]"=0, "Initialize array[60]"=0, "Initialize array[61]"=0, "Initialize array[62]"=0, "Initialize array[63]"=0}} ("TCANFD"), "AIdxchn"=w127, "AId"="CH1ID", "AIsStd"="CH1 Frame Format", "AIsData"="CH1 Frame Type", "ADLC"="CANFD DLC", "AIsFD"="CH1  FD Frame", "FDatas"=w133, "BRS"="BRS") -> (w134:T4)
            n77 = disable-structure shown="启用" {
              disable-tunnel: w134 -> [w139 _]
              disable-tunnel: w131 -> [w138 _]
              frame Enabled {
                n78 = call "tsapp_transmit_canfd_async.vi"("TCANFD"=w139, "Path"=w138) -> ()  [unwired: 7 in, 3 out]
              }
              frame Disabled {
              }
            }
          }
        }
        n79 = local read "Exit"() -> (w125:bool)
      }
      n80 = while {
        shift-right: [w103] -> _
        shift-left: _ -> [w104]
        stop <- w106 stop-if-true
        # "CANFD2Read"
        n81 = local read "Hardware on/off"() -> (w102:bool)
        n82 = local read "Enable CH2"() -> (w100:bool)
        n83 = Wait (ms)(milliseconds to wait=u32 100 ("等待时间（毫秒）")) -> ()  [unwired: 1 out]
        n84 = And(x=w102, y=w100) -> (x .and. y?=w101:bool)
        n85 = case shown="真" w101 {
          tunnel: [w107 w112] -> w103
          tunnel: w104 -> [w107 w116]
          frame False {
            (unwired) T6 [] ("数组")
          }
          frame True {
            n86 = local read "CH2 Application Logic Channel"() -> (w110:i32)
            n87 = call "TSCAN_GetDllPath.vi"() -> ("DllPath"=w113:path)  [unwired: 11 in]
            n88 = call "tsfifo_receive_canfd_msgs.vi"("Display message type"="CH2 Display Message Type", "AAPPChannel"=w110, "Path"=w113) -> ("ACANMsgBuffer"=w108:T7)  [unwired: 4 in, 3 out]
            n89 = Insert Into Array(array=w116, new element=w108) -> (w114:T7)  [unwired: 1 in]
            n90 = Array Size(array=w114) -> (size(s)=w115:i32)
            n91 = case shown="300.." w115 {
              selector: w115 -> [_ w122]
              tunnel: [w117 w120] -> w112
              tunnel: w114 -> [w117 w118]
              frame 0, Default {
              }
              frame 300.. {
                n92 = Subtract(x=w122, y=300) -> (x-y=w119:i32)
                n93 = Array Subset(array=w118, index=w119) -> (w120:T7)  [unwired: 1 in]
              }
            }
            n94 = control-ref of="CH2Data"() -> (w111:refnum<vi>)
            n95 = call "TSCANfd_Table.vi"("Messages"=w112, "MCListbox reference handle"=w111) -> ()  [unwired: 10 in]
          }
        }
        n96 = local read "Exit"() -> (w106:bool)
      }
      n97 = while {
        stop <- w87 stop-if-true
        # "CANFD2Write"
        n98 = Wait (ms)(milliseconds to wait=u32 100 ("等待时间（毫秒）")) -> ()  [unwired: 1 out]
        n99 = case shown="真" "CH2 Sending" {
          frame False {
          }
          frame True {
            n100 = local read "CH2 Physical Channel"() -> (w98:i32)
            n101 = call "TSCAN_GetDllPath.vi"() -> ("DllPath"=w99:path)  [unwired: 11 in]
            n102 = Array To Cluster(array="CH2SendData") -> (cluster=w92:T11)
            n103 = Bundle By Name(cluster=T4 {"AIdxchn"=0, "AId"=0, "AIsStd"=0, "BRS"=enum."Close", "AIsData"=0, "ADLC"=0, "AIsFD"=enum."Classic CAN Message", "FDatas"={"Initialize array[0]"=0, "Initialize array[1]"=0, "Initialize array[2]"=0, "Initialize array[3]"=0, "Initialize array[4]"=0, "Initialize array[5]"=0, "Initialize array[6]"=0, "Initialize array[7]"=0, "Initialize array[8]"=0, "Initialize array[9]"=0, "Initialize array[10]"=0, "Initialize array[11]"=0, "Initialize array[12]"=0, "Initialize array[13]"=0, "Initialize array[14]"=0, "Initialize array[15]"=0, "Initialize array[16]"=0, "Initialize array[17]"=0, "Initialize array[18]"=0, "Initialize array[19]"=0, "Initialize array[20]"=0, "Initialize array[21]"=0, "Initialize array[22]"=0, "Initialize array[23]"=0, "Initialize array[24]"=0, "Initialize array[25]"=0, "Initialize array[26]"=0, "Initialize array[27]"=0, "Initialize array[28]"=0, "Initialize array[29]"=0, "Initialize array[30]"=0, "Initialize array[31]"=0, "Initialize array[32]"=0, "Initialize array[33]"=0, "Initialize array[34]"=0, "Initialize array[35]"=0, "Initialize array[36]"=0, "Initialize array[37]"=0, "Initialize array[38]"=0, "Initialize array[39]"=0, "Initialize array[40]"=0, "Initialize array[41]"=0, "Initialize array[42]"=0, "Initialize array[43]"=0, "Initialize array[44]"=0, "Initialize array[45]"=0, "Initialize array[46]"=0, "Initialize array[47]"=0, "Initialize array[48]"=0, "Initialize array[49]"=0, "Initialize array[50]"=0, "Initialize array[51]"=0, "Initialize array[52]"=0, "Initialize array[53]"=0, "Initialize array[54]"=0, "Initialize array[55]"=0, "Initialize array[56]"=0, "Initialize array[57]"=0, "Initialize array[58]"=0, "Initialize array[59]"=0, "Initialize array[60]"=0, "Initialize array[61]"=0, "Initialize array[62]"=0, "Initialize array[63]"=0}} ("TCANFD"), "AIdxchn"=w98, "AId"="CH2ID", "AIsStd"="CH2 Frame Format", "AIsData"="CH2 Frame Type", "ADLC"="CANFD DLC 2", "AIsFD"="CH2  FD Frame", "FDatas"=w92, "BRS"="BRS 2") -> (w88:T4)
            n104 = call "tsapp_transmit_canfd_async.vi"("TCANFD"=w88, "Path"=w99) -> ()  [unwired: 7 in, 3 out]
          }
        }
        n105 = local read "Exit"() -> (w87:bool)
      }
      n106 = while {
        shift-right: [w65] -> _
        shift-left: _ -> [w66]
        stop <- w68 stop-if-true
        # "CANFD3Read"
        n107 = local read "Hardware on/off"() -> (w64:bool)
        n108 = local read "Enable CH3"() -> (w63:bool)
        n109 = Wait (ms)(milliseconds to wait=u32 100 ("等待时间（毫秒）")) -> ()  [unwired: 1 out]
        n110 = And(x=w64, y=w63) -> (x .and. y?=w62:bool)
        n111 = case shown="真" w62 {
          tunnel: [w69 w74] -> w65
          tunnel: w66 -> [w69 w78]
          frame False {
            (unwired) T6 [] ("数组")
          }
          frame True {
            n112 = local read "CH3 Application Logic Channel"() -> (w73:i32)
            n113 = call "TSCAN_GetDllPath.vi"() -> ("DllPath"=w75:path)  [unwired: 11 in]
            n114 = call "tsfifo_receive_canfd_msgs.vi"("Display message type"="CH3 Display Message Type", "AAPPChannel"=w73, "Path"=w75) -> ("ACANMsgBuffer"=w70:T7)  [unwired: 4 in, 3 out]
            n115 = Insert Into Array(array=w78, new element=w70) -> (w76:T7)  [unwired: 1 in]
            n116 = Array Size(array=w76) -> (size(s)=w77:i32)
            n117 = case shown="300.." w77 {
              selector: w77 -> [_ w84]
              tunnel: [w79 w82] -> w74
              tunnel: w76 -> [w79 w80]
              frame 0, Default {
              }
              frame 300.. {
                n118 = Subtract(x=w84, y=300) -> (x-y=w81:i32)
                n119 = Array Subset(array=w80, index=w81) -> (w82:T7)  [unwired: 1 in]
              }
            }
            n120 = control-ref of="CH3Data"() -> (w71:refnum<vi>)
            n121 = call "TSCANfd_Table.vi"("Messages"=w74, "MCListbox reference handle"=w71) -> ()  [unwired: 10 in]
          }
        }
        n122 = local read "Exit"() -> (w68:bool)
      }
      n123 = while {
        stop <- w49 stop-if-true
        # "CANFD3 Write"
        n124 = Wait (ms)(milliseconds to wait=u32 100 ("等待时间（毫秒）")) -> ()  [unwired: 1 out]
        n125 = case shown="真" "CH3 Sending" {
          frame False {
          }
          frame True {
            n126 = local read "CH3 Physical Channel"() -> (w60:i32)
            n127 = call "TSCAN_GetDllPath.vi"() -> ("DllPath"=w61:path)  [unwired: 11 in]
            n128 = Array To Cluster(array="CH3SendData") -> (cluster=w54:T12)
            n129 = Bundle By Name(cluster=T4 {"AIdxchn"=0, "AId"=0, "AIsStd"=0, "BRS"=enum."Close", "AIsData"=0, "ADLC"=0, "AIsFD"=enum."Classic CAN Message", "FDatas"={"Initialize array[0]"=0, "Initialize array[1]"=0, "Initialize array[2]"=0, "Initialize array[3]"=0, "Initialize array[4]"=0, "Initialize array[5]"=0, "Initialize array[6]"=0, "Initialize array[7]"=0, "Initialize array[8]"=0, "Initialize array[9]"=0, "Initialize array[10]"=0, "Initialize array[11]"=0, "Initialize array[12]"=0, "Initialize array[13]"=0, "Initialize array[14]"=0, "Initialize array[15]"=0, "Initialize array[16]"=0, "Initialize array[17]"=0, "Initialize array[18]"=0, "Initialize array[19]"=0, "Initialize array[20]"=0, "Initialize array[21]"=0, "Initialize array[22]"=0, "Initialize array[23]"=0, "Initialize array[24]"=0, "Initialize array[25]"=0, "Initialize array[26]"=0, "Initialize array[27]"=0, "Initialize array[28]"=0, "Initialize array[29]"=0, "Initialize array[30]"=0, "Initialize array[31]"=0, "Initialize array[32]"=0, "Initialize array[33]"=0, "Initialize array[34]"=0, "Initialize array[35]"=0, "Initialize array[36]"=0, "Initialize array[37]"=0, "Initialize array[38]"=0, "Initialize array[39]"=0, "Initialize array[40]"=0, "Initialize array[41]"=0, "Initialize array[42]"=0, "Initialize array[43]"=0, "Initialize array[44]"=0, "Initialize array[45]"=0, "Initialize array[46]"=0, "Initialize array[47]"=0, "Initialize array[48]"=0, "Initialize array[49]"=0, "Initialize array[50]"=0, "Initialize array[51]"=0, "Initialize array[52]"=0, "Initialize array[53]"=0, "Initialize array[54]"=0, "Initialize array[55]"=0, "Initialize array[56]"=0, "Initialize array[57]"=0, "Initialize array[58]"=0, "Initialize array[59]"=0, "Initialize array[60]"=0, "Initialize array[61]"=0, "Initialize array[62]"=0, "Initialize array[63]"=0}} ("TCANFD"), "AIdxchn"=w60, "AId"="CH3ID", "AIsStd"="CH3 Frame Format", "AIsData"="CH3 Frame Type", "ADLC"="CANFD DLC 3", "AIsFD"="CH3 FD Frame", "FDatas"=w54, "BRS"="BRS 3") -> (w50:T4)
            n130 = call "tsapp_transmit_canfd_async.vi"("TCANFD"=w50, "Path"=w61) -> ()  [unwired: 7 in, 3 out]
          }
        }
        n131 = local read "Exit"() -> (w49:bool)
      }
      n132 = while {
        shift-right: [w27] -> _
        shift-left: _ -> [w28]
        stop <- w30 stop-if-true
        # "CANFD4Read"
        n133 = local read "Hardware on/off"() -> (w26:bool)
        n134 = local read "Enable CH4"() -> (w24:bool)
        n135 = Wait (ms)(milliseconds to wait=u32 100 ("等待时间（毫秒）")) -> ()  [unwired: 1 out]
        n136 = And(x=w26, y=w24) -> (x .and. y?=w25:bool)
        n137 = case shown="真" w25 {
          tunnel: [w31 w36] -> w27
          tunnel: w28 -> [w31 w40]
          frame False {
            (unwired) T6 [] ("数组")
          }
          frame True {
            n138 = local read "CH4 Application Logic Channel"() -> (w35:i32)
            n139 = call "TSCAN_GetDllPath.vi"() -> ("DllPath"=w37:path)  [unwired: 11 in]
            n140 = call "tsfifo_receive_canfd_msgs.vi"("Display message type"="CH4 Display Message Type", "AAPPChannel"=w35, "Path"=w37) -> ("ACANMsgBuffer"=w32:T7)  [unwired: 4 in, 3 out]
            n141 = Insert Into Array(array=w40, new element=w32) -> (w38:T7)  [unwired: 1 in]
            n142 = Array Size(array=w38) -> (size(s)=w39:i32)
            n143 = case shown="300.." w39 {
              selector: w39 -> [_ w46]
              tunnel: [w41 w44] -> w36
              tunnel: w38 -> [w41 w42]
              frame 0, Default {
              }
              frame 300.. {
                n144 = Subtract(x=w46, y=300) -> (x-y=w43:i32)
                n145 = Array Subset(array=w42, index=w43) -> (w44:T7)  [unwired: 1 in]
              }
            }
            n146 = control-ref of="CH4Data"() -> (w33:refnum<vi>)
            n147 = call "TSCANfd_Table.vi"("Messages"=w36, "MCListbox reference handle"=w33) -> ()  [unwired: 10 in]
          }
        }
        n148 = local read "Exit"() -> (w30:bool)
      }
      n149 = while {
        stop <- w11 stop-if-true
        # "CANFD4Write"
        n150 = Wait (ms)(milliseconds to wait=u32 100 ("等待时间（毫秒）")) -> ()  [unwired: 1 out]
        n151 = case shown="真" "CH4 Sending" {
          frame False {
          }
          frame True {
            n152 = local read "CH4 Physical Channel"() -> (w22:i32)
            n153 = call "TSCAN_GetDllPath.vi"() -> ("DllPath"=w23:path)  [unwired: 11 in]
            n154 = Array To Cluster(array="CH4SendData") -> (cluster=w16:T13)
            n155 = Bundle By Name(cluster=T4 {"AIdxchn"=0, "AId"=0, "AIsStd"=0, "BRS"=enum."Close", "AIsData"=0, "ADLC"=0, "AIsFD"=enum."Classic CAN Message", "FDatas"={"Initialize array[0]"=0, "Initialize array[1]"=0, "Initialize array[2]"=0, "Initialize array[3]"=0, "Initialize array[4]"=0, "Initialize array[5]"=0, "Initialize array[6]"=0, "Initialize array[7]"=0, "Initialize array[8]"=0, "Initialize array[9]"=0, "Initialize array[10]"=0, "Initialize array[11]"=0, "Initialize array[12]"=0, "Initialize array[13]"=0, "Initialize array[14]"=0, "Initialize array[15]"=0, "Initialize array[16]"=0, "Initialize array[17]"=0, "Initialize array[18]"=0, "Initialize array[19]"=0, "Initialize array[20]"=0, "Initialize array[21]"=0, "Initialize array[22]"=0, "Initialize array[23]"=0, "Initialize array[24]"=0, "Initialize array[25]"=0, "Initialize array[26]"=0, "Initialize array[27]"=0, "Initialize array[28]"=0, "Initialize array[29]"=0, "Initialize array[30]"=0, "Initialize array[31]"=0, "Initialize array[32]"=0, "Initialize array[33]"=0, "Initialize array[34]"=0, "Initialize array[35]"=0, "Initialize array[36]"=0, "Initialize array[37]"=0, "Initialize array[38]"=0, "Initialize array[39]"=0, "Initialize array[40]"=0, "Initialize array[41]"=0, "Initialize array[42]"=0, "Initialize array[43]"=0, "Initialize array[44]"=0, "Initialize array[45]"=0, "Initialize array[46]"=0, "Initialize array[47]"=0, "Initialize array[48]"=0, "Initialize array[49]"=0, "Initialize array[50]"=0, "Initialize array[51]"=0, "Initialize array[52]"=0, "Initialize array[53]"=0, "Initialize array[54]"=0, "Initialize array[55]"=0, "Initialize array[56]"=0, "Initialize array[57]"=0, "Initialize array[58]"=0, "Initialize array[59]"=0, "Initialize array[60]"=0, "Initialize array[61]"=0, "Initialize array[62]"=0, "Initialize array[63]"=0}} ("TCANFD"), "AIdxchn"=w22, "AId"="CH4ID", "AIsStd"="CH4 Frame Format", "AIsData"="CH4 Frame Type", "ADLC"="CANFD DLC 4", "AIsFD"="CH4  FD Frame", "FDatas"=w16, "BRS"="BRS 4") -> (w12:T4)
            n156 = call "tsapp_transmit_canfd_async.vi"("TCANFD"=w12, "Path"=w23) -> ()  [unwired: 7 in, 3 out]
          }
        }
        n157 = local read "Exit"() -> (w11:bool)
      }
    }
  }
